vi "FX15.vi"(11 "Variables and Memory in":T1 {"GFX" format="%02x"}) -> (3 "Variables and Memory out":T1 {"GFX" format="%02x"})   [LabVIEW 2021]
uses:
  Controls/ClusterF.ctl
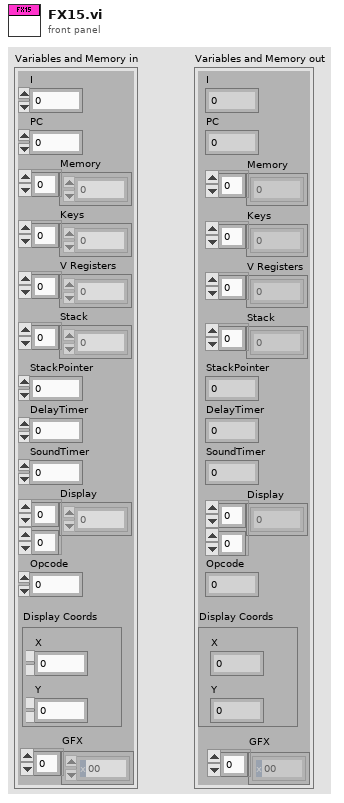
[diagram p1: front panel]
types:
  T1 = typedef "ClusterF.ctl" = cluster{"I":u16, "PC":u16, "Memory":u8[], "Keys":u8[], "V Registers":u8[], "Stack":u16[], "StackPointer":u16, "DelayTimer":u8, "SoundTimer":u8, "Display":u8[][], "Opcode":u16, "Display Coords":cluster{"X":u8, "Y":u8}, "GFX":u8[]}
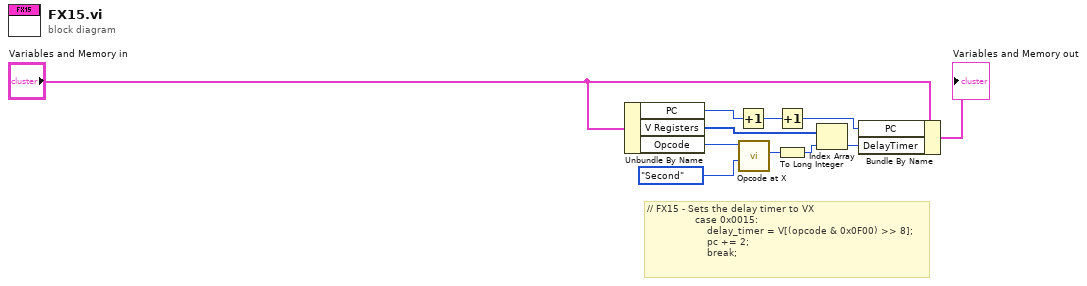
[diagram p0: block diagram]
diagram:
  # "// FX15 - Sets the delay timer to VX\n                case 0x0015:\n                    delay_timer = V[(opcode & 0x0F00) >> 8];\n                    pc += 2;\n                    break;"
  n1 = Unbundle By Name("Variables and Memory in") -> ("PC"=w3:u16, "V Registers"=w8:u8[], "Opcode"=w6:u16)
  n2 = Increment(x=w3) -> (x+1=w4:u16)
  n3 = call "Opcode at X.vi"("X Position"=enum16{"First", "Second", "Third", "Fourth"}."Second", "Opcode"=w6) -> ("Opcode at X Position (U8)"=w9:u8)  [unwired: 9 in]
  n4 = Increment(x=w4) -> (x+1=w5:u16)
  n5 = To Long Integer(number=w9) -> (32bit integer=w10:i32)
  n6 = Index Array(array=w8, index=w10) -> (element=w11:u8)
  n7 = Bundle By Name(cluster="Variables and Memory in", "PC"=w5, "DelayTimer"=w11) -> (→"Variables and Memory out":T1)
